vi "Write Sub Exports.vi"(8 "error in (no error)":errorcluster, 10 "Sub Installers":variant, 11 "NSIS_Installer in":refnum<class "Compound_Installer.lvclass">) -> (0 "error out":errorcluster, 3 "NSIS_Installer out":refnum<class "Compound_Installer.lvclass">)   [LabVIEW 2017, in "CL_G3_VIComponentBuilder.lvlib" / "Compound_Installer.lvclass"]
uses:
  Compound_Installer.lvclass
  Compound_Installer.lvclass/Compound_Installer.ctl
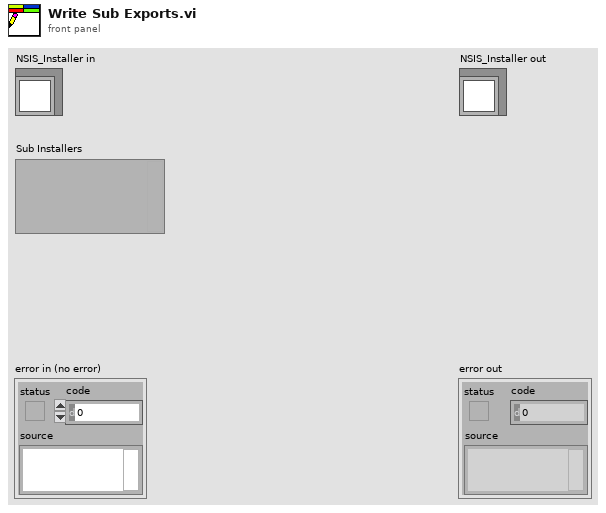
[diagram p1: front panel]
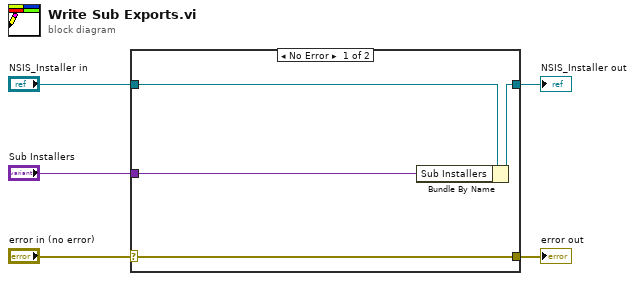
[diagram p0: block diagram]
diagram:
  n1 = case shown="No Error" "error in (no error)" {
    selector: "error in (no error)" -> [w9 w10]
    tunnel: [w9 w10] -> w4
    tunnel: [w7 w11] -> w2
    tunnel: "NSIS_Installer in" -> [w8 w11]
    tunnel: "Sub Installers" -> [w6 _]
    frame No Error {
      n2 = Bundle By Name(cluster=w8, "Sub Installers"=w6) -> (w7:refnum<class "Compound_Installer.lvclass">)
    }
    frame Error {
    }
  }
  "error out" <- w4
  "NSIS_Installer out" <- w2
